vi "Read Multiple Measurements (Voltage Data).vi"(0 "VISA resource name":refnum<visa-resource-name>, 5 "Maximum Time (30000 ms)":i32=30000, 11 "error in (no error)":errorcluster) -> (4 "VISA resource name out":refnum<visa-resource-name>, 6 "Instantaneous Voltage":dbl[](array[numeric]), 8 "Voltage Harmonic Amplitudes":dbl[](array[numeric]), 10 "Voltage Harmonic Phase Angles":dbl[](array[numeric]), 15 "error out":errorcluster)   [LabVIEW 2019, in "Agilent 681x Series.lvlib"]
doc: "Initiates and reads 4096 instantaneous voltage measurements, the first 50 current harmonic amplitudes and phase values.\n\n<B>Note:</B>\n\nThis VI changes the <B>Trigger Source</B> to <B>Bus</B> and uses a software trigger after the instrument is initiated. If you want to control the triggering and other features, please use the low level VIs."
uses:
  <instrlib>/Agilent 681x Series/Agilent 681x Series.lvlib
  <instrlib>/Agilent 681x Series/Public/Data/Low Level/Fetch Multiple Measurements (Voltage Data).vi
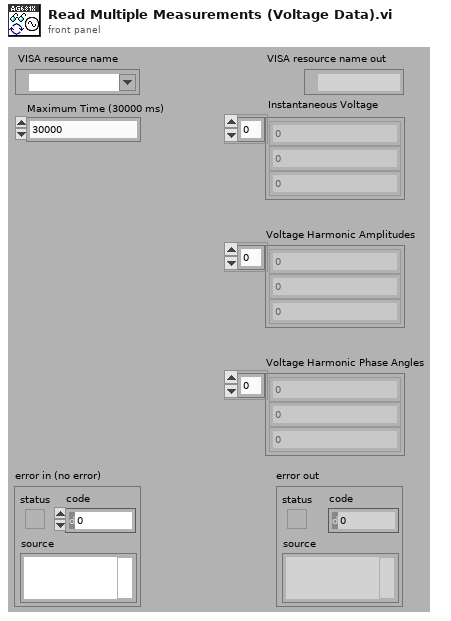
[diagram p1: front panel]
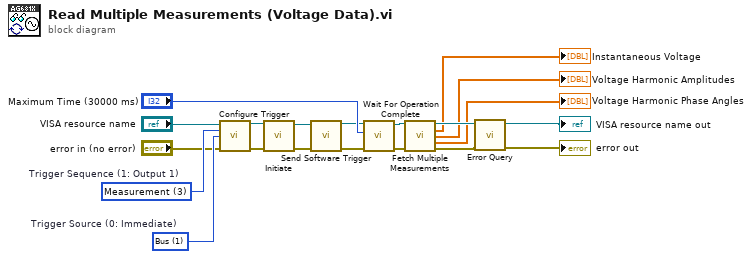
[diagram p0: block diagram]
diagram:
  w16 = 1 items=["Immediate", "Bus", "External", "Phase", "Trigger Out"]  # Trigger Source (0: Immediate)
  w17 = 3 items=["Output"=1, "Synchronous Source"=2, "Measurement"=3]  # Trigger Sequence (1: Output 1)
  n1 = call <instrlib>:"Configure Trigger.vi"("VISA resource name"="VISA resource name", "Trigger Sequence (1: Output 1)"=w17, "Trigger Source (0: Immediate)"=w16, "error in (no error)"="error in (no error)") -> ("VISA resource name out"=w14:refnum<visa-resource-name>, "error out"=w15:errorcluster)  [unwired: 10 in]
  n2 = call <instrlib>:"Initiate.vi"("error in (no error)"=w15, "VISA resource name"=w14) -> ("error out"=w13:errorcluster, "VISA resource name out"=w12:refnum<visa-resource-name>)  [unwired: 8 in]
  n3 = call <instrlib>:"Send Software Trigger.vi"("VISA resource name"=w12, "error in (no error)"=w13) -> ("VISA resource name out"=w10:refnum<visa-resource-name>, "error out"=w11:errorcluster)  [unwired: 12 in]
  n4 = call <instrlib>:"Wait For Operation Complete.vi"("error in (no error)"=w11, "Maximum Time (10000 ms)"="Maximum Time (30000 ms)", "VISA resource name"=w10) -> ("error out"=w18:errorcluster, "VISA resource name out"=w19:refnum<visa-resource-name>)  [unwired: 7 in]
  n5 = call-poly <instrlib>:"Fetch Multiple Measurements.vi"("VISA resource name"=w19, "error in (no error)"=w18) -> ("VISA resource name out"=w7:refnum<visa-resource-name>, "Instantaneous Voltage"=→"Instantaneous Voltage":dbl[], "Voltage Harmonic Amplitudes"=→"Voltage Harmonic Amplitudes":dbl[], "Voltage Harmonic Phase Angles"=→"Voltage Harmonic Phase Angles":dbl[], "error out"=w6:errorcluster)  [unwired: 9 in]
  n6 = call <instrlib>:"Error Query.vi"("error in (no error)"=w6, "VISA resource name"=w7) -> ("error out"=→"error out":errorcluster, "VISA resource name out"=→"VISA resource name out":refnum<visa-resource-name>)  [unwired: 6 in, 2 out]
